vi "Puntje 5 stoppen.vi"() -> ()   [LabVIEW 2019]
panel:
  out "Wat moet de auto doen?":string="Stoppen"
  in  "Array":dbl[](array[numeric])
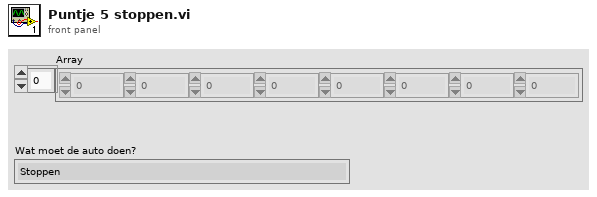
[diagram p1: front panel]
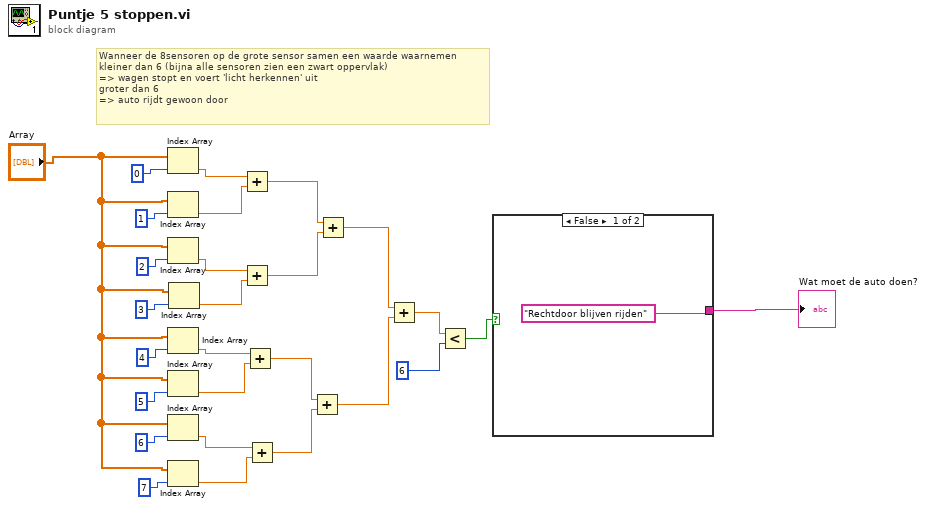
[diagram p0: block diagram]
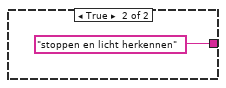
[diagram p2: hidden frame]
diagram:
  # "Wanneer de 8sensoren op de grote sensor samen een waarde waarnemen \nkleiner dan 6 (bijna alle sensoren zien een zwart oppervlak) \n=> wagen stopt en voert 'licht herkennen' uit\ngroter dan 6 \n=> auto rijdt gewoon door"
  n1 = Index Array(array="Array", index=0) -> (element=w18:dbl)
  n2 = Index Array(array="Array", index=1) -> (element=w17:dbl)
  n3 = Index Array(array="Array", index=2) -> (element=w16:dbl)
  n4 = Index Array(array="Array", index=4) -> (element=w14:dbl)
  n5 = Index Array(array="Array", index=5) -> (element=w13:dbl)
  n6 = Index Array(array="Array", index=6) -> (element=w12:dbl)
  n7 = Index Array(array="Array", index=7) -> (element=w11:dbl)
  n8 = Index Array(array="Array", index=3) -> (element=w15:dbl)
  n9 = Add(x=w18, y=w17) -> (x+y=w7:dbl)
  n10 = Add(x=w16, y=w15) -> (x+y=w8:dbl)
  n11 = Add(x=w14, y=w13) -> (x+y=w9:dbl)
  n12 = Add(x=w12, y=w11) -> (x+y=w10:dbl)
  n13 = Add(x=w9, y=w10) -> (x+y=w5:dbl)
  n14 = Add(x=w7, y=w8) -> (x+y=w6:dbl)
  n15 = Add(x=w6, y=w5) -> (x+y=w4:dbl)
  n16 = Less?(x=w4, y=6) -> (x < y?=w1:bool)
  n17 = case shown="False" w1 {
    tunnel: ["Rechtdoor blijven rijden" "stoppen en licht herkennen"] -> w2
    frame False {
    }
    frame True {
    }
  }
  "Wat moet de auto doen?" <- w2
